vi "Folders Cleanup.vi"(8 "error in (no error)":errorcluster) -> (0 "error out":errorcluster)   [LabVIEW 2013]
uses:
  Global Variables/General Globals.vi
panel:
  out "Files & folders":i32
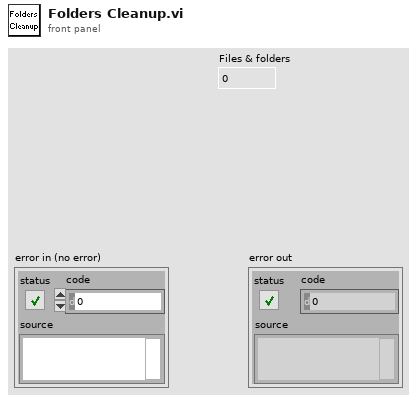
[diagram p1: front panel]
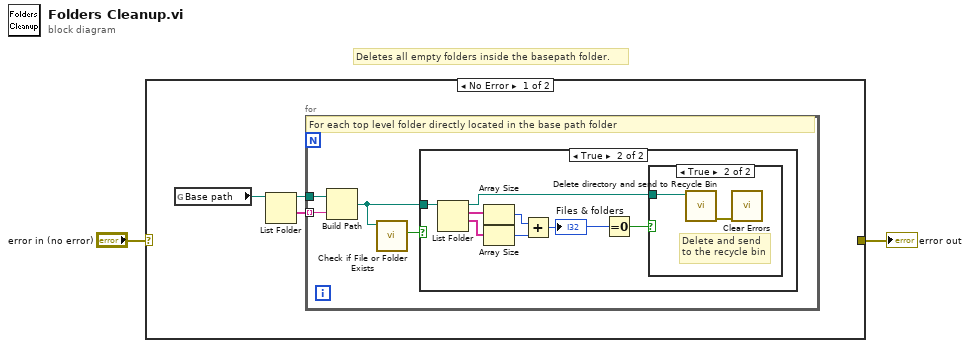
[diagram p0: block diagram]
diagram:
  # "Deletes all empty folders inside the basepath folder."
  n1 = case shown="No Error" "error in (no error)" {
    selector: "error in (no error)" -> [_ w20]
    tunnel: [_ w20] -> w1
    frame No Error {
      n2 = global read "General Globals.vi" "Base path"() -> (w4:path)
      n3 = List Folder(path=w4) -> (path out=w5:path, folder names=w3:string[])  [unwired: 3 in, 2 out]
      n4 = for {
        tunnel: w5 -> [w9]
        tunnel: w3 -> [w6] mode=indexing
        # "For each top level folder directly located in the base path folder"
        n5 = Build Path(base path=w9, name or relative path=w6) -> (appended path=w8:path)
        n6 = call <vilib>:"Check if File or Folder Exists.vi"("path"=w8) -> ("file or folder exists?"=w7:bool)  [unwired: 8 in, 2 out]
        n7 = case shown="True" w7 {
          tunnel: w8 -> [_ w17]
          frame False {
          }
          frame True {
            n8 = List Folder(path=w17) -> (path out=w10:path, filenames=w16:string[], folder names=w15:string[])  [unwired: 3 in, 1 out]
            n9 = Array Size(array=w16) -> (size(s)=w14:i32)
            n10 = Array Size(array=w15) -> (size(s)=w13:i32)
            n11 = Add(x=w14, y=w13) -> (x+y=w12:i32)
            "Files & folders" <- w12
            n12 = Equal To 0?(x=w12) -> (x = 0?=w11:bool)
            n13 = case shown="True" w11 {
              tunnel: w10 -> [_ w19]
              frame False {
              }
              frame True {
                # "Delete and send to the recycle bin"
                n14 = call "Delete directory and send to Recycle Bin.vi"("Directory to Recycle"=w19) -> ("error out"=w18:errorcluster)  [unwired: 10 in]
                n15 = call <vilib>:"Clear Errors.vi"("error in (no error)"=w18) -> ()  [unwired: 6 in, 1 out]
              }
            }
          }
        }
      }
    }
    frame Error {
    }
  }
  "error out" <- w1
